vi "NI_FPGA_PPG.publish cmd data description.vi"(0 "i ref in":refnum<vi>, 2 "cmd_data_string":string, 3 "ms timeout (10000)":i32=10000, 5 "error in (no error)":errorcluster) -> (14 "i ref out":refnum<vi>, 17 "timed out":bool, 19 "error out":errorcluster)   [LabVIEW 2014, in "NI_FPGA_PPG.lvlib"]
doc: "Publishes a string with the last (pattern-)command received from the host.\n\nLicense Agreement for this software:\n\nCopyright (C) 2009\nFalk Ziegler\nInstitut für Physik\nErnst-Moritz-Arndt Universität\nFelix-Hausdorff-Str. 6\n17487 Greifswald\n\nContact: Falk Ziegler, ziegler@physik.uni-greifswald.de\n\nThis program is free software: you can redistribute it and/or modify it under the terms of the GNU General Public License as published by the Free Software Foundation, either version 3 of the License, or (at your option) any later version.\n\nThis program is distributed in the hope that it will be useful, but WITHOUT ANY WARRANTY; without even the implied warranty of MERCHANTABILITY or FITNESS FOR A PARTICULAR PURPOSE. See the GNU General Public License for more details.\n\nYou should have received a copy of the GNU General Public License along with this program. If not, see <http://www.gnu.org/licenses/>.\n\nFor all questions and ideas contact: ziegler@physik.uni-greifswald.de or d.beck@gsi.de\nLast update: 01-Sep-2009"
uses:
  NI_FPGA_PPG.lvlib
  CSlibraries-extern/DimLVEvent/LVDimInterface/LVDimInterface.lvlib
  CS_Core/CSSystem/CSSystemLib/CSSystemLib.lvlib
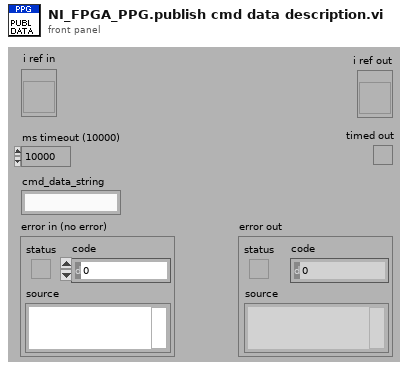
[diagram p1: front panel]
types:
  T1 = typedef "NI_FPGA_PPG.lvlib/NI_FPGA_PPG.i attribute.ctl" = cluster{"dim_service_id":cluster{"dim_actual_device_status":i32, "dim_event_data":i32, "dim_cmd_data":i32, "dim_cmd_data _description":i32, "dim_channel_description":i32}, "VISA":refnum<visa-resource-name>, "actual_device_status":i32, "event_data_id":i32, "pdc_enabled":bool, "pdc_timestamp":u32, "cmd_data_string":string, "cmd_data_size":i32, "cmd_data_description_string":string, "cmd_data_description_size":i32, "channel_description_string":string, "channel_description_size":i32}
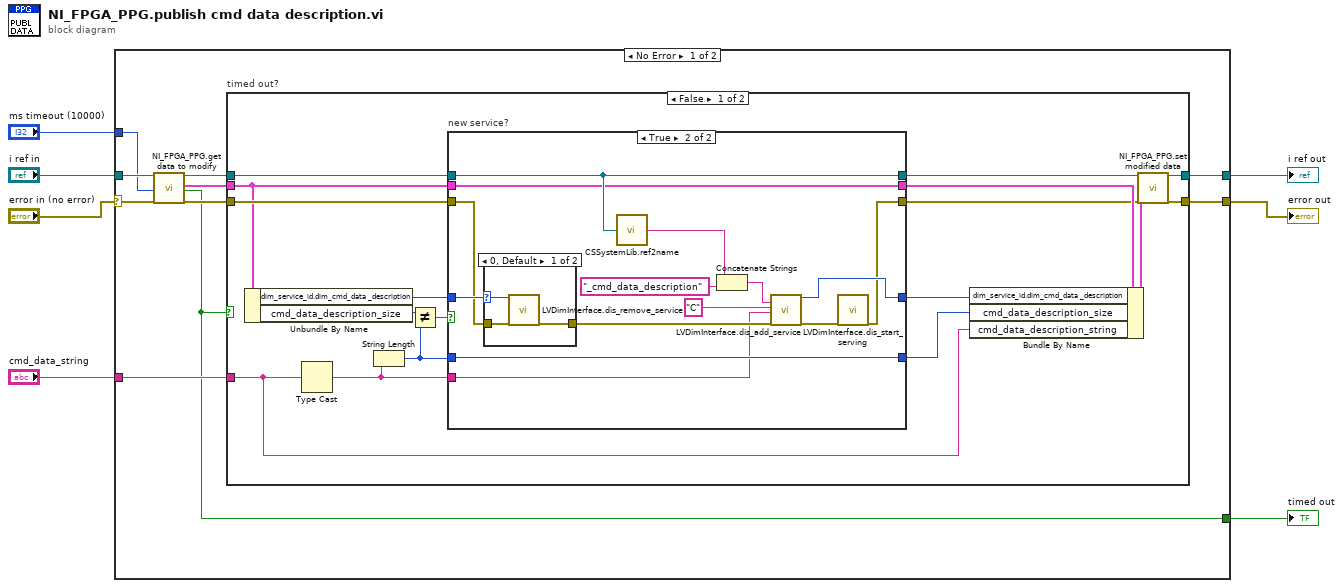
[diagram p0: block diagram]
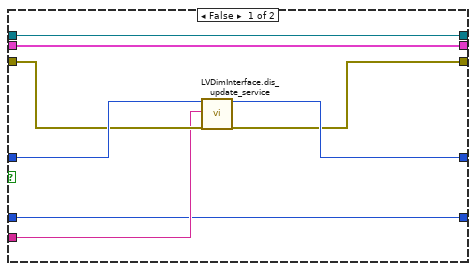
[diagram p2: hidden frame]
diagram:
  n1 = case shown="No Error" "error in (no error)" {
    selector: "error in (no error)" -> [w14 w62]
    tunnel: "i ref in" -> [w16 w63]
    tunnel: [w17 w63] -> w5
    tunnel: [w9 w62] -> w4
    tunnel: "ms timeout (10000)" -> [w11 _]
    tunnel: "cmd_data_string" -> [w10 _]
    tunnel: [w8 _] -> w1
    frame No Error {
      n2 = call "NI_FPGA_PPG.get data to modify.vi"("i ref in"=w16, "ms timeout (10000)"=w11, "error in (no error)"=w14) -> ("i ref out"=w15:refnum<vi>, "i attribute"=w12:T1, "timed out"=w8:bool, "error out"=w13:errorcluster)  [unwired: 13 in]
      n3 = case "timed out?" shown="False" w8 {
        tunnel: [w28 w61] -> w17
        tunnel: w15 -> [w31 w61]
        tunnel: w13 -> [w30 w60]
        tunnel: w12 -> [w27 _]
        tunnel: w10 -> [w18 _]
        tunnel: [w20 w60] -> w9
        frame False {
          n4 = Unbundle By Name(w27) -> ("dim_service_id.dim_cmd_data _description"=w32:i32, "cmd_data_description_size"=w33:i32)
          n5 = Type Cast(x=w18) -> (*(type *) &x=w19:string)  [unwired: 1 in]
          n6 = String Length(string=w19) -> (length=w22:i32)
          n7 = Not Equal?(x=w33, y=w22) -> (x != y?=w34:bool)
          n8 = case "new service?" shown="True" w34 {
            tunnel: w31 -> [w42 w51]
            tunnel: [w42 w51] -> w29
            tunnel: w32 -> [w41 w56]
            tunnel: w30 -> [w40 w52]
            tunnel: w19 -> [w37 w46]
            tunnel: [w39 w50] -> w25
            tunnel: [w38 w49] -> w24
            tunnel: w27 -> [w35 w48]
            tunnel: [w35 w48] -> w26
            tunnel: w22 -> [w36 w47]
            tunnel: [w36 w47] -> w21
            frame False {
              n9 = call "LVDimInterface.dis_update_service.vi"("my_serviceID"=w41, "data"=w37, "error in (no error)"=w40) -> ("my_serviceID out"=w39:i32, "error out"=w38:errorcluster)  [unwired: 14 in, 1 out]
            }
            frame True {
              n10 = case shown="0, Default" w56 {
                selector: w56 -> [w59 _]
                tunnel: [w58 _] -> w55
                tunnel: w52 -> [w57 _]
                frame 0, Default {
                  n11 = call "LVDimInterface.dis_remove_service.vi"("my_serviceID"=w59, "error in (no error)"=w57) -> ("error out"=w58:errorcluster)  [unwired: 17 in]
                }
                frame -1 {
                }
              }
              n12 = call "CSSystemLib.ref2name.vi"("obj refnum"=w51) -> ("name"=w44:string)
              n13 = Concatenate Strings(w44, "_cmd_data_description" ("string")) -> (w43:string)
              n14 = call "LVDimInterface.dis_add_service.vi"("serviceName"=w43, "typeDescriptor"="C", "data"=w46, "error in (no error)"=w55) -> ("my_serviceID"=w50:i32, "error out"=w53:errorcluster)  [unwired: 14 in]
              n15 = call "LVDimInterface.dis_start_serving.vi"("error in (no error)"=w53) -> ("error out"=w49:errorcluster)  [unwired: 17 in, 1 out]
            }
          }
          n16 = Bundle By Name(cluster=w26, "dim_service_id.dim_cmd_data _description"=w25, "cmd_data_description_size"=w21, "cmd_data_description_string"=w18) -> (w23:T1)
          n17 = call "NI_FPGA_PPG.set modified data.vi"("i ref in"=w29, "i attribute"=w23, "error in (no error)"=w24) -> ("i ref out"=w28:refnum<vi>, "error out"=w20:errorcluster)  [unwired: 15 in]
        }
        frame True {
        }
      }
    }
    frame Error {
    }
  }
  "error out" <- w4
  "i ref out" <- w5
  "timed out" <- w1
